vi "Get Window Image.vi"(8 "error in (no error)":errorcluster, 10 "subset rect":T2, 11 "Ctl Ref":refnum<vi>) -> (0 "error out":errorcluster, 1 "Ctl Portion Picture":picture, 2 "Ctl Portion Image Data":T1, 3 "Ctl Ref out":refnum<vi>)   [LabVIEW 2020, in "MacroAssert.lvlib"]
uses:
  MacroAssert.lvlib
  <vilib>/picture/picture.llb/imagedata.ctl
  <vilib>/Utility/miscctls.llb/LVPointTypeDef.ctl
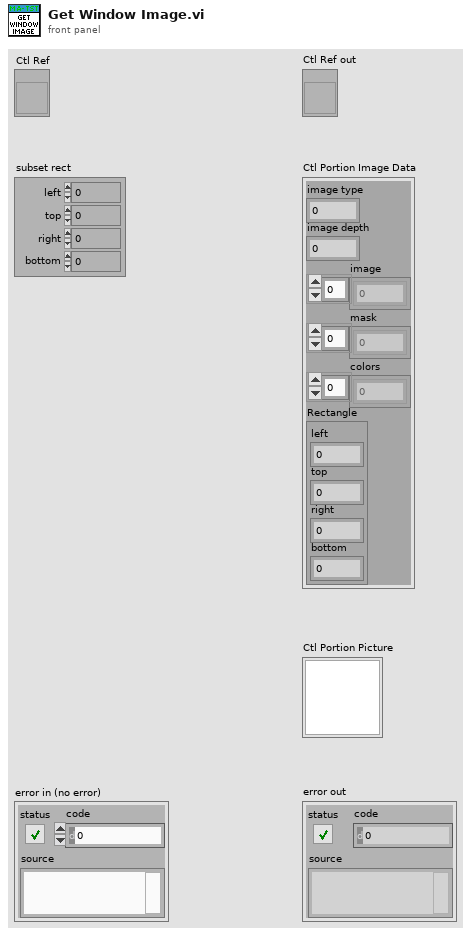
[diagram p1: front panel]
types:
  T1 = typedef "imagedata.ctl" = cluster{"image type":i32, "image depth":i32, "image":u8[], "mask":u8[], "colors":u32[], "Rectangle":cluster{"left":i16, "top":i16, "right":i16, "bottom":i16}}
  T2 = cluster{"left":i16, "top":i16, "right":i16, "bottom":i16}
  T3 = typedef "LVPointTypeDef.ctl" = cluster{"Horizontal":i16, "Vertical":i16}
  T4 = typedef "LVRectTypeDef.ctl" = cluster{"Left":i16, "Top":i16, "Right":i16, "Bottom":i16}
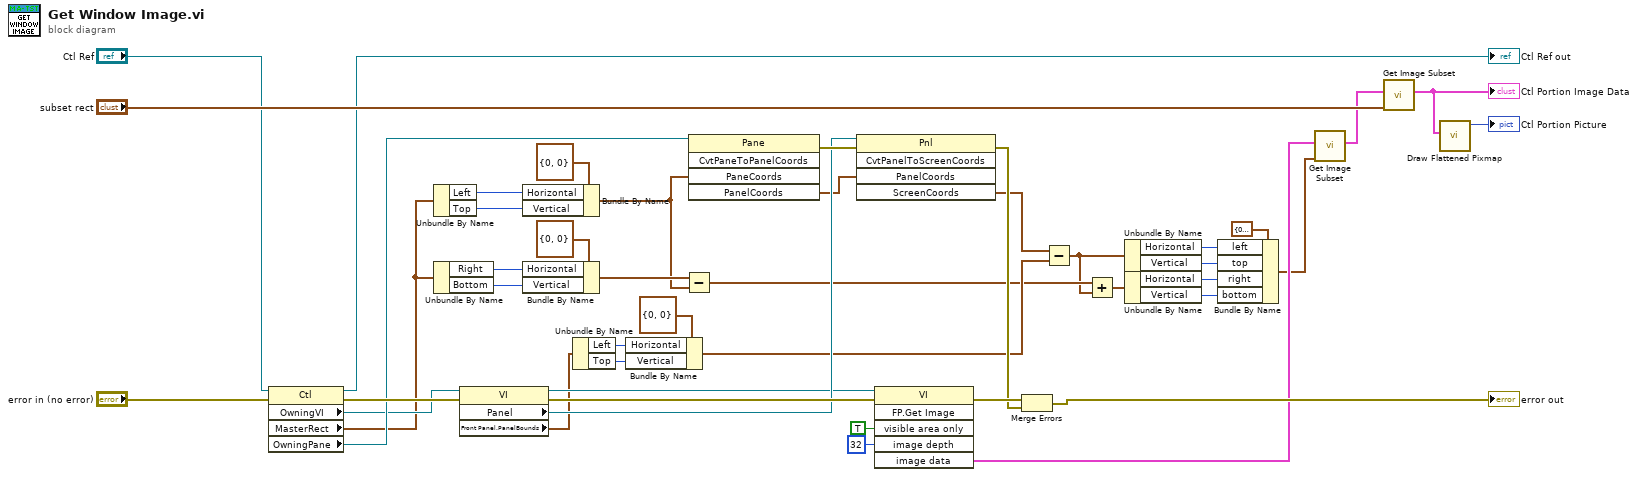
[diagram p0: block diagram]
diagram:
  n1 = property class="Ctl"(reference="Ctl Ref", error in="error in (no error)") -> (reference out=→"Ctl Ref out":refnum<vi>, error out=w43:errorcluster, "OwningVI"=w26:refnum<vi>, "MasterRect"=w18:T4, "OwningPane"=w32:refnum<vi>)
  n2 = Unbundle By Name(w18) -> ("Left"=w30:i16, "Top"=w29:i16)
  n3 = Unbundle By Name(w18) -> ("Right"=w16:i16, "Bottom"=w15:i16)
  n4 = property class="VI"(reference=w26, error in=w43) -> (reference out=w3:refnum<vi>, error out=w41:errorcluster, "Panel"=w25:refnum<vi>, "Front Panel.PanelBounds"=w2:T4)
  n5 = Bundle By Name(cluster=T3 {"Horizontal"=0, "Vertical"=0} ("Pane Coordinates"), "Horizontal"=w30, "Vertical"=w29) -> (w13:T3)
  n6 = Bundle By Name(cluster=T3 {"Horizontal"=0, "Vertical"=0} ("Pane Coordinates"), "Horizontal"=w16, "Vertical"=w15) -> (w14:T3)
  n7 = Unbundle By Name(w2) -> ("Left"=w21:i16, "Top"=w20:i16)
  n8 = Bundle By Name(cluster=T3 {"Horizontal"=0, "Vertical"=0} ("Pane Coordinates"), "Horizontal"=w21, "Vertical"=w20) -> (w19:T3)
  n9 = Subtract(x=w14, y=w13) -> (x-y=w11:T3)
  n10 = invoke class="Pane" method="CvtPaneToPanelCoords"(reference=w32, "PaneCoords"=w13) -> (error out=w42:errorcluster, "PanelCoords"=w24:T3)  [unwired: 3 in, 3 out]
  n11 = invoke class="Pnl" method="CvtPanelToScreenCoords"(reference=w25, error in=w42, "PanelCoords"=w24) -> (error out=w39:errorcluster, "ScreenCoords"=w23:T3)  [unwired: 2 in, 3 out]
  n12 = invoke class="VI" method="FP.Get Image"(reference=w3, error in=w41, "visible area only"=TRUE ("Visible Area Only"), "image depth"=32 ("Image Depth")) -> (error out=w44:errorcluster, "image data"=w27:T1)  [unwired: 2 in, 4 out]
  n13 = Merge Errors(w44, w39) -> (→"error out":errorcluster)
  n14 = Subtract(x=w23, y=w19) -> (x-y=w10:T3)
  n15 = Add(x=w11, y=w10) -> (x+y=w7:T3)
  n16 = Unbundle By Name(w10) -> ("Horizontal"=w9:i16, "Vertical"=w8:i16)
  n17 = Unbundle By Name(w7) -> ("Horizontal"=w6:i16, "Vertical"=w5:i16)
  n18 = Bundle By Name(cluster=T2 {"left"=0, "top"=0, "right"=0, "bottom"=0} ("subset rect"), "left"=w9, "top"=w8, "right"=w6, "bottom"=w5) -> (w4:T2)
  n19 = call <vilib>:"Get Image Subset.vi"("subset rect"=w4, "image data"=w27) -> ("image subset"=w28:T1)  [unwired: 4 in, 1 out]
  n20 = call <vilib>:"Get Image Subset.vi"("subset rect"="subset rect", "image data"=w28) -> ("image subset"=w37:T1)  [unwired: 4 in, 1 out]
  "Ctl Portion Image Data" <- w37
  n21 = call <vilib>:"Draw Flattened Pixmap.vi"("image data"=w37) -> ("new picture"=→"Ctl Portion Picture":picture)  [unwired: 8 in]
